vi "Log L1.vi"(8 "error in (no error)":errorcluster, 10 "Array":waveform(dbl)[](array[waveform]), 11 "Logging Configuration":T1) -> (0 "error out":errorcluster)   [LabVIEW 2014, in "PLS Logging.lvlib"]
uses:
  PLS Logging.lvlib
  Logging Configuration.ctl
  reshape debit.vi
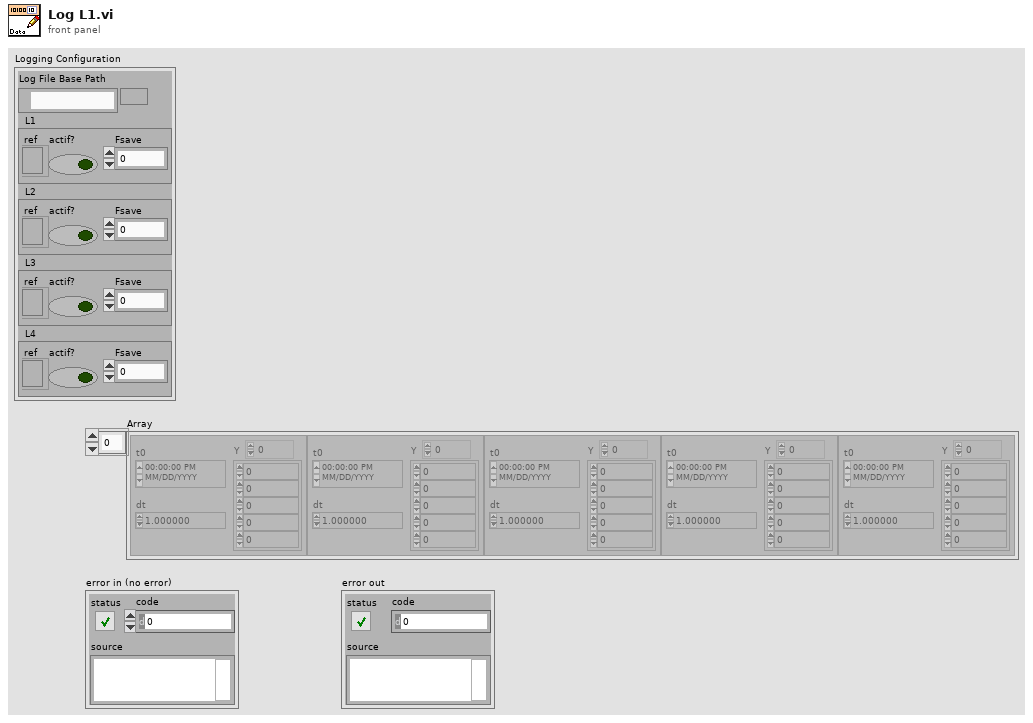
[diagram p1: front panel]
types:
  T1 = typedef "PLS Logging.lvlib/Logging Configuration.ctl" = cluster{"Log File Base Path":path, "L1":cluster{"ref":refnum<file>, "actif?":bool, "Fsave":dbl}, "L2":cluster{"ref":refnum<file>, "actif?":bool, "Fsave":dbl}, "L3":cluster{"ref":refnum<file>, "actif?":bool, "Fsave":dbl}, "L4":cluster{"ref":refnum<file>, "actif?":bool, "Fsave":dbl}}
  T2 = cluster{"ref":refnum<file>, "actif?":bool, "Fsave":dbl}
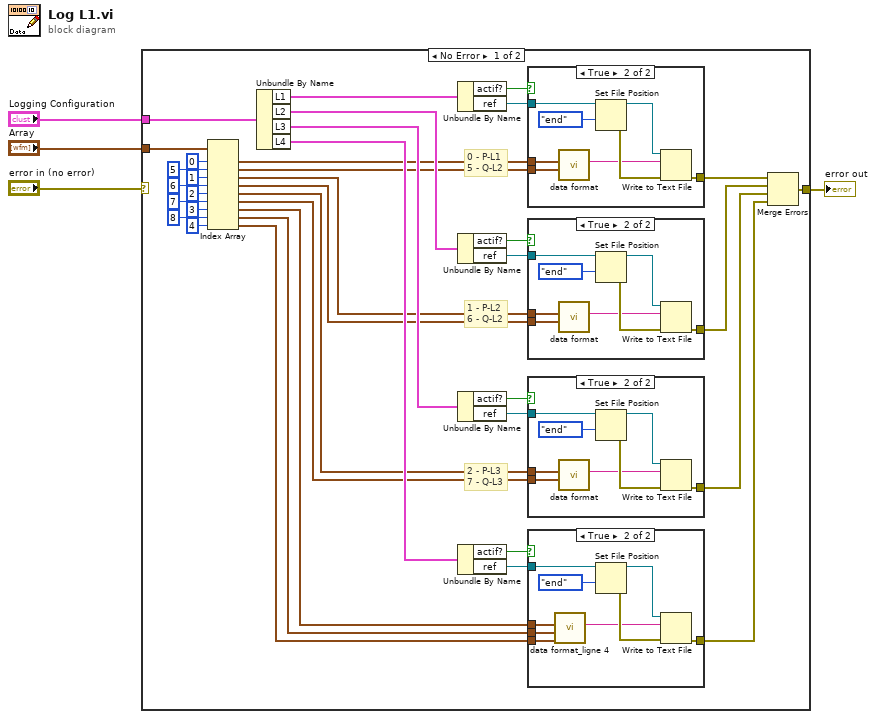
[diagram p0: block diagram]
diagram:
  n1 = case shown="No Error" "error in (no error)" {
    selector: "error in (no error)" -> [_ w75]
    tunnel: "Array" -> [w41 _]
    tunnel: "Logging Configuration" -> [w39 _]
    tunnel: [w35 w75] -> w2
    frame No Error {
      # "2 - P-L3\n7 - Q-L3"
      # "1 - P-L2\n6 - Q-L2"
      # "0 - P-L1\n5 - Q-L2"
      n2 = Index Array(array=w41, index #1=0 ("index"), index #2=5 ("index"), index #3=1 ("index"), index #4=6 ("index"), index #5=2 ("index"), index #6=7 ("index"), index #7=3 ("index"), index #8=8 ("index"), index #9=4 ("index")) -> (element #1=w13:waveform(dbl), element #2=w12:waveform(dbl), element #3=w11:waveform(dbl), element #4=w10:waveform(dbl), element #5=w9:waveform(dbl), element #6=w8:waveform(dbl), element #7=w7:waveform(dbl), element #8=w6:waveform(dbl), element #9=w5:waveform(dbl))
      n3 = Unbundle By Name(w39) -> ("L1"=w38:T2, "L2"=w32:T2, "L3"=w26:T2, "L4"=w25:T2)
      n4 = Unbundle By Name(w38) -> ("actif?"=w37:bool, "ref"=w36:refnum<file>)
      n5 = Unbundle By Name(w32) -> ("actif?"=w33:bool, "ref"=w34:refnum<file>)
      n6 = Unbundle By Name(w26) -> ("actif?"=w27:bool, "ref"=w28:refnum<file>)
      n7 = Unbundle By Name(w25) -> ("actif?"=w30:bool, "ref"=w29:refnum<file>)
      n8 = case shown="True" w37 {
        tunnel: [_ w74] -> w40
        tunnel: w36 -> [_ w72]
        tunnel: w13 -> [_ w68]
        tunnel: w12 -> [_ w67]
        frame False {
        }
        frame True {
          n9 = call "data format.vi"("Q"=w67, "P"=w68) -> ("spreadsheet string"=w69:string)  [unwired: 9 in]
          n10 = Set File Position(refnum=w72, from (0:start)=enum16{"start", "end", "current"}."end") -> (refnum out=w71:refnum<file>, error out=w70:errorcluster)  [unwired: 2 in]
          n11 = Write to Text File(file (use dialog)=w71, text=w69, error in=w70) -> (error out=w74:errorcluster)  [unwired: 1 in, 2 out]
        }
      }
      n12 = case shown="True" w33 {
        tunnel: [_ w66] -> w31
        tunnel: w34 -> [_ w64]
        tunnel: w11 -> [_ w60]
        tunnel: w10 -> [_ w59]
        frame False {
        }
        frame True {
          n13 = call "data format.vi"("Q"=w59, "P"=w60) -> ("spreadsheet string"=w61:string)  [unwired: 9 in]
          n14 = Set File Position(refnum=w64, from (0:start)=enum16{"start", "end", "current"}."end") -> (refnum out=w63:refnum<file>, error out=w62:errorcluster)  [unwired: 2 in]
          n15 = Write to Text File(file (use dialog)=w63, text=w61, error in=w62) -> (error out=w66:errorcluster)  [unwired: 1 in, 2 out]
        }
      }
      n16 = case shown="True" w27 {
        tunnel: [_ w58] -> w24
        tunnel: w28 -> [_ w56]
        tunnel: w9 -> [_ w52]
        tunnel: w8 -> [_ w51]
        frame False {
        }
        frame True {
          n17 = call "data format.vi"("Q"=w51, "P"=w52) -> ("spreadsheet string"=w53:string)  [unwired: 9 in]
          n18 = Set File Position(refnum=w56, from (0:start)=enum16{"start", "end", "current"}."end") -> (refnum out=w55:refnum<file>, error out=w54:errorcluster)  [unwired: 2 in]
          n19 = Write to Text File(file (use dialog)=w55, text=w53, error in=w54) -> (error out=w58:errorcluster)  [unwired: 1 in, 2 out]
        }
      }
      n20 = case shown="True" w30 {
        tunnel: w29 -> [_ w48]
        tunnel: [_ w50] -> w23
        tunnel: w7 -> [_ w44]
        tunnel: w6 -> [_ w43]
        tunnel: w5 -> [_ w42]
        frame False {
        }
        frame True {
          n21 = call "data format_ligne 4.vi"("T"=w42, "Q"=w43, "P"=w44) -> ("spreadsheet string"=w45:string)  [unwired: 8 in]
          n22 = Set File Position(refnum=w48, from (0:start)=enum16{"start", "end", "current"}."end") -> (refnum out=w47:refnum<file>, error out=w46:errorcluster)  [unwired: 2 in]
          n23 = Write to Text File(file (use dialog)=w47, text=w45, error in=w46) -> (error out=w50:errorcluster)  [unwired: 1 in, 2 out]
        }
      }
      n24 = Merge Errors(w40, w31, w24, w23) -> (w35:errorcluster)
    }
    frame Error {
    }
  }
  "error out" <- w2
